vi "Read Mod enc.vi"(9 "invert":bool, 11 "Mod Ref":string) -> (1 "rot angle":dbl, 2 "SWERVE_DRIVE_MODULE_STATE":T3 {"Angle"."SIN" format="%13.4f"; "Angle"."COS" format="%13.4f"; "Angle"."VALUE" format="%13.4f"}, 3 "SWERVE_DRIVE_MODULE_POSITION":T1 {"Angle"."SIN" format="%13.4f"; "Angle"."COS" format="%13.4f"; "Angle"."VALUE" format="%13.4f"})   [LabVIEW 2020]
doc: "Vi to Read the Encoders of Our 2023 swerve modules . Returns Module state and Position"
uses:
  <vilib>/Rock Robotics/WPI/ThirdParty/JAS_Junk/TrajLib/TypeDef/SWERVE_DRIVE_MODULE_STATE.ctl
  <vilib>/Rock Robotics/WPI/ThirdParty/JAS_Junk/TrajLib/TypeDef/ROTATION2D.ctl
  <vilib>/Rock Robotics/WPI/ThirdParty/JAS_Junk/TrajLib/TypeDef/SWERVE_DRIVE_MODULE_POSITION.ctl
  <vilib>/Rock Robotics/WPI/ThirdParty/JAS_Junk/TrajLib/Trajectory_Library.lvlib
panel:
  out "Sensor Velocity":dbl
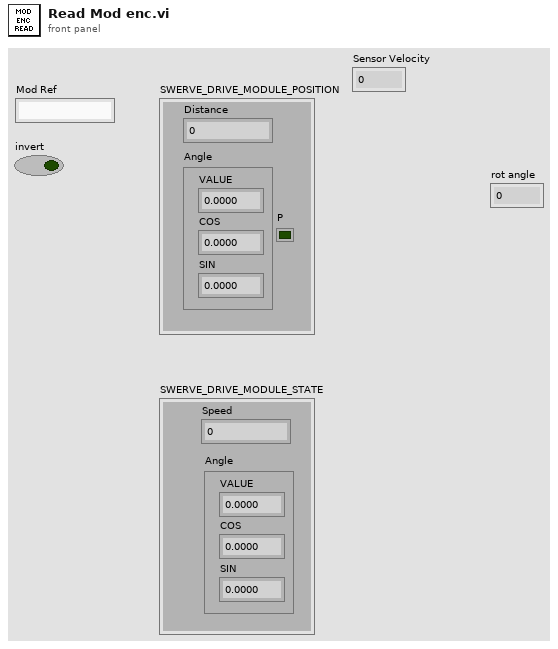
[diagram p1: front panel]
types:
  T1 = typedef "Trajectory_Library.lvlib/SWERVE_DRIVE_MODULE_POSITION.ctl" = cluster{"Distance":dbl, "Angle":T2, "P":bool}
  T2 = typedef "Trajectory_Library.lvlib/ROTATION2D.ctl" = cluster{"VALUE":dbl, "COS":dbl, "SIN":dbl}
  T3 = typedef "Trajectory_Library.lvlib/SWERVE_DRIVE_MODULE_STATE.ctl" = cluster{"Speed":dbl, "Angle":T2}
  T4 = typedef "WPI_MotorControlDeviceRef.ctl" = cluster{"DeviceStatus":errorcluster, "Type":T5, "PWM":cluster{"PWM Channel":T6, "DeadBand":T7}, "CAN":cluster{"Device Number":u8, "SetOutput VI Ref":variant, "GetOutput VI Ref":variant, "Enable VI Ref":variant, "Disable VI Ref":variant, "Data":variant}, "Invert":bool, "DIO PWM":cluster{"PWM \"Enable\" Channel":T6, "DIOChannel":T8, "PWM Rate":dbl}}
  T5 = typedef "WPI_MotorControlType.ctl" = enum16{"PWM", "CAN", "DIO PWM"}
  T6 = typedef "FPGA_DIOPWMChannel.ctl" = enum8{"PWM 0", "PWM 1", "PWM 2", "PWM 3", "PWM 4", "PWM 5", "PWM 6", "PWM 7", "PWM 8", "PWM 9", "PWM MXP 0", "PWM MXP 1", "PWM MXP 2", "PWM MXP 3", "PWM MXP 4", "PWM MXP 5", "PWM MXP 6", "PWM MXP 7", "PWM MXP 8", "PWM MXP 9", "Invalid"}
  T7 = typedef "WPI_PWMDeadband.ctl" = cluster{"Name":string, "maxPositivePwm":i32, "minPositivePwm":i32, "centerPwm":i32, "maxNegativePwm":i32, "minNegativePwm":i32, "angularRange":u16}
  T8 = typedef "FPGA_DIOChannel.ctl" = enum8{"DIO 0", "DIO 1", "DIO 2", "DIO 3", "DIO 4", "DIO 5", "DIO 6", "DIO 7", "DIO 8", "DIO 9", "DIO MXP 0", "DIO MXP 1", "DIO MXP 2", "DIO MXP 3", "DIO MXP 4", "DIO MXP 5", "DIO MXP 6", "DIO MXP 7", "DIO MXP 8", "DIO MXP 9", "DIO MXP 10", "DIO MXP 11", "DIO MXP 12", "DIO MXP 13", "DIO MXP 14", "DIO MXP 15", "SPI Port CS1", "SPI Port CS2", "SPI Port CS3", "SPI Port MISO", "SPI Port MOSI", "Invalid"}
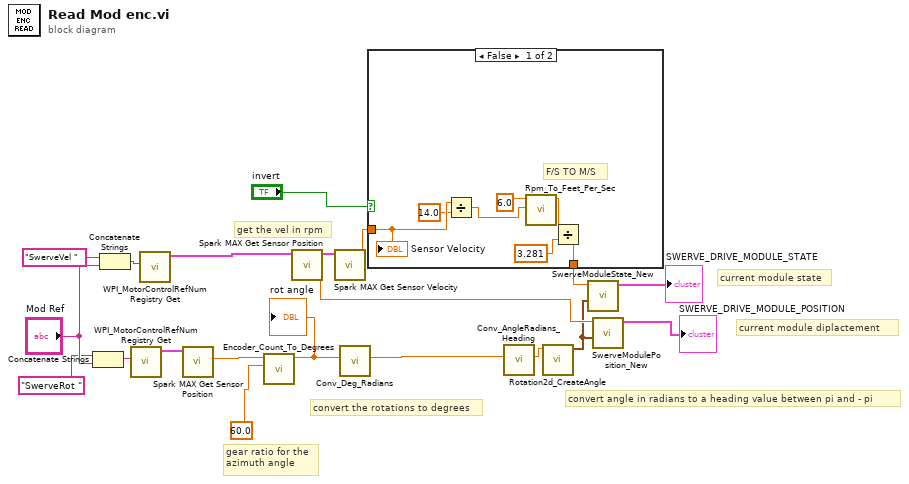
[diagram p0: block diagram]
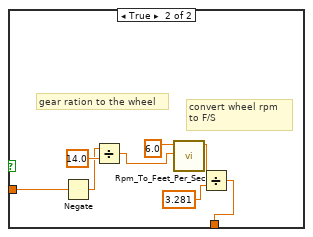
[diagram p2: hidden frame]
diagram:
  # "current module diplactement"
  # "current module state"
  # "get the vel in rpm"
  # "convert angle in radians to a heading value between pi and - pi"
  # "convert the rotations to degrees"
  # "gear ratio for the \nazimuth angle"
  n1 = Concatenate Strings("SwerveRot " ("refnum name"), "Mod Ref") -> (w19:string)
  n2 = Concatenate Strings("SwerveVel " ("refnum name"), "Mod Ref") -> (w18:string)
  n3 = call <vilib>:"WPI_MotorControlRefNum Registry Get.vi"("refnum name"=w19) -> ("MotorControlDevRef"=w7:T4)  [unwired: 9 in, 1 out]
  n4 = call <vilib>:"WPI_MotorControlRefNum Registry Get.vi"("refnum name"=w18) -> ("MotorControlDevRef"=w9:T4)  [unwired: 9 in, 1 out]
  n5 = call <vilib>:"Spark MAX Get Sensor Position.vi"("MotorControlDevRef in"=w7) -> ("Sensor Position"=w6:dbl)  [unwired: 7 in, 3 out]
  n6 = call "Encoder_Count_To_Degrees.vi"("Counts per Rev"=60.0 ("y"), "Sensor Position"=w6) -> ("Degrees"=w4:dbl)  [unwired: 9 in]
  "rot angle" <- w4
  n7 = call <vilib>:"Spark MAX Get Sensor Position.vi"("MotorControlDevRef in"=w9) -> ("Sensor Position"=w13:dbl, "MotorControlDevRef out"=w10:T4)  [unwired: 7 in, 2 out]
  n8 = call <vilib>:"Spark MAX Get Sensor Velocity.vi"("MotorControlDevRef in"=w10) -> ("Sensor Velocity"=w2:dbl)  [unwired: 7 in, 3 out]
  n9 = call <vilib>:"Conv_Deg_Radians.vi"("Degress"=w4) -> ("Radians"=w8:dbl)  [unwired: 10 in]
  n10 = case shown="False" "invert" {
    tunnel: [w25 w30] -> w3
    tunnel: w2 -> [w23 w29]
    frame False {
      # "F/S TO M/S"
      n11 = Divide(x=w23, y=14.0) -> (x/y=w22:dbl)
      n12 = call "Rpm_To_Feet_Per_Sec.vi"("RPM"=w22, "Diameter"=6.0) -> ("Numeric"=w26:dbl)  [unwired: 9 in]
      n13 = Divide(x=w26, y=3.281) -> (x/y=w25:dbl)
      "Sensor Velocity" <- w23
    }
    frame True {
      # "convert wheel rpm \nto F/S"
      # "gear ration to the wheel"
      n14 = Negate(x=w29) -> (-x=w28:dbl)
      n15 = Divide(x=w28, y=14.0) -> (x/y=w32:dbl)
      n16 = call "Rpm_To_Feet_Per_Sec.vi"("RPM"=w32, "Diameter"=6.0) -> ("Numeric"=w34:dbl)  [unwired: 9 in]
      n17 = Divide(x=w34, y=3.281) -> (x/y=w30:dbl)
    }
  }
  n18 = call <vilib>:"Conv_AngleRadians_Heading.vi"("Radians"=w8) -> ("Heading"=w11:dbl)  [unwired: 10 in]
  n19 = call <vilib>:"Rotation2d_CreateAngle.vi"("Angle"=w11) -> ("ROTATION"=w12:T2)  [unwired: 10 in]
  n20 = call <vilib>:"SwerveModuleState_New.vi"("ROTATION"=w12, "Speed"=w3) -> ("SWERVE_DRIVE_MODULE_STATE"=→"SWERVE_DRIVE_MODULE_STATE":T3)  [unwired: 9 in]
  n21 = call <vilib>:"SwerveModulePosition_New.vi"("ROTATION"=w12, "Distance"=w13) -> ("SWERVE_DRIVE_MODULE_POSITION"=→"SWERVE_DRIVE_MODULE_POSITION":T1)  [unwired: 9 in]
